vi "gds_top_tx.vi"(0 "Modulation Parameters":T2={"TX Parameters"={"Sampling Rate"=1000000.0, "Oversample Factor"=2}, "Shared Parameters"={"Packet Length"=500, "Preamble Length"=20, "modulation type"=enum."OOK", "FSK deviation (Hz)"=625.0, "Filter Parameters"={"modulation type"=enum."ASK", "pulse shaping filter (none)"=enum."none", "filter length (symbols)"=8, "filter parameter"=0.5}}}, 5 "HW parameters In":T3={"Device IP Address"="192.168.10.26", "Active Antenna"="TX1", "Carrier Frequency (Hz)"=433001000.0, "Gain (dB)"=20.0, "Generation Mode"=enum."continuous"} {"Gain (dB)" format="%.2f"; "Carrier Frequency (Hz)" format="%.2p"}, 7 "STOP":bool, 11 "error in":errorcluster) -> (1 "Transmitting":bool, 2 "coerced carrier frequency (Hz)":dbl format="%#_6p", 3 "coerced gain (dB)":dbl format="%#_6f", 4 "Modulation Parameters Out":T2, 6 "HW parameters out":T3={"Device IP Address"="192.168.11.3", "Active Antenna"="TX1", "Carrier Frequency (Hz)"=915000000.0, "Gain (dB)"=10.0, "Generation Mode"=enum."continuous"} {"Gain (dB)" format="%.2f"; "Carrier Frequency (Hz)" format="%.2p"}, 8 "key bit sequence":i8[](array[numeric])=[0, 0, 0, 0, 0, 0, 0, 0, 1, 1, 1, 0, 1, 0, 0, 1, 1, 0, 1, 1, 1, 0, 0, 1, 0, 0, 0, 1, 0, 1, 0, 0, 0, 0, 1, 0, 1, 0, 1, 1, 0, 1, 0, 0, 1, 1, 1, 1, 1, 1, 0, 1, 1, 0, 0, 1, 0, 0, 1, 0, 0, 1, 0, 1, 1, 0, 1, 1, 1, 1, 1, 1, 0, 0, 1, 0, 0, 1, 1, 0, 1, 0, 1, 0, 0, 1, 1, 0, 0, 1, 1, 0, 0, 0, 0, 0, 0, 0, 1, 1, 0, 0, 0, 1, 1, 0, 0, 1, 0, 1, 0, 0, 0, 1, 1, 0, 1, 0, 0, 1, 0, 1, 1, 1, 1, 1, 1, 1, 0, 1, 0, 0, 0, 1, 0, 1, 1, 0, 0, 0, 1, 1, 1, 0, 1, 0, 1, 1, 0, 0, 1, 0, 1, 1, 0, 0, 1, 1, 1, 1, 0, 0, 0, 1, 1, 1, 1, 1, 0, 1, 1, 1, 0, 1, 0, 0, 0, 0, 0, 1, 1, 0, 1, 0, 1, 1, 0, 1, 1, 0, 1, 1, 1, 0, 1, 1, 0, 0, 0, 0, 0, 1, 0, 1, 1, 0, 1, 0, 1, 1, 1, 1, 1, 0, 1, 0, 1, 0, 1, 0, 1, 0, 0, 0, 0, 0, 0, 1, 0, 1, 0, 0, 1, 0, 1, 0, 1, 1, 1, 1, 0, 0, 1, 0, 1, 1, 1, 0, 1, 1, 1, 0, 0, 0, 0, 0, 0, 1, 1, 1, 0, 0, 1, 1, 1, 0, 1, 0, 0, 1, 0, 0, 1, 1, 1, 1, 0, 1, 0, 1, 1, 1, 0, 1, 0, 1, 0, 0, 0, 1, 0, 0, 1, 0, 0, 0, 0, 1, 1, 0, 0, 1, 1, 1, 0, 0, 0, 0, 1, 0, 1, 1, 1, 1, 0, 1, 1, 0, 1, 1, 0, 0, 1, 1, 0, 1, 0, 0, 0, 0, 1, 1, 1, 0, 1, 1, 1, 1, 0, 0, 0, 0, 1, 1, 1, 1, 1, 1, 1, 1, 1, 0, 0, 0, 0, 0, 1, 1, 1, 1, 0, 1, 1, 1, 1, 1, 0, 0, 0, 1, 0, 1, 1, 1, 0, 0, 1, 1, 0, 0, 1, 0, 0, 0, 0, 0, 1, 0, 0, 1, 0, 1, 0, 0, 1, 1, 1, 0, 1, 1, 0, 1, 0, 0, 0, 1, 1, 1, 1, 0, 0, 1, 1, 1, 1, 1, 0, 0, 1, 1, 0, 1, 1, 0, 0, 0, 1, 0, 1, 0, 1, 0, 0, 1, 0, 0, 0, 1, 1, 1, 0, 0, 0, 1, 1, 0, 1, 1, 0, 1, 0, 1, 0, 1, 1, 1, 0, 0, 0, 1, 0, 0, 1, 1, 0, 0, 0, 1, 0, 0, 0, 1, 0, 0, 0, 0, 0, 0, 0, 0, 1, 0, 0, 0, 0, 1, 0, 0, 0, 1, 1, 0, 0, 0, 0, 1, 0, 0, 1, 1], 10 "output IQ waveform":cluster{"t0":dbl, "dt":dbl, "Y":cdb[]}, 12 "packet duration (sec)":dbl min=50000000.0 max=100000000.0 step=50000000.0 format="%#_6p", 13 "symbol rate (Hz)":dbl min=50000000.0 max=100000000.0 step=50000000.0 format="%#_6p", 14 "data symbols":cdb[](array[numeric])=[0.0+0.0i, 0.7071067811865475+0.7071067811865475i, -0.7071067811865475-0.7071067811865475i, 0.7071067811865475-0.7071067811865475i, -0.7071067811865475-0.7071067811865475i, -0.7071067811865475+0.7071067811865475i, -0.7071067811865475+0.7071067811865475i, 0.7071067811865475-0.7071067811865475i, -0.7071067811865475+0.7071067811865475i, -0.7071067811865475-0.7071067811865475i, -0.7071067811865475+0.7071067811865475i, 0.7071067811865475-0.7071067811865475i, 0.7071067811865475+0.7071067811865475i, 0.7071067811865475-0.7071067811865475i, 0.7071067811865475-0.7071067811865475i, 0.7071067811865475+0.7071067811865475i, 0.7071067811865475+0.7071067811865475i, -0.7071067811865475+0.7071067811865475i, -0.7071067811865475+0.7071067811865475i, -0.7071067811865475-0.7071067811865475i, 0.7071067811865475-0.7071067811865475i, 0.7071067811865475+0.7071067811865475i, -0.7071067811865475-0.7071067811865475i, -0.7071067811865475-0.7071067811865475i, -0.7071067811865475-0.7071067811865475i, 0.7071067811865475-0.7071067811865475i, -0.7071067811865475+0.7071067811865475i, 0.7071067811865475-0.7071067811865475i, 0.7071067811865475+0.7071067811865475i, -0.7071067811865475+0.7071067811865475i, 0.7071067811865475-0.7071067811865475i, 0.7071067811865475-0.7071067811865475i, -0.7071067811865475+0.7071067811865475i, -0.7071067811865475-0.7071067811865475i, -0.7071067811865475-0.7071067811865475i, -0.7071067811865475-0.7071067811865475i, 0.7071067811865475+0.7071067811865475i, -0.7071067811865475+0.7071067811865475i, 0.7071067811865475-0.7071067811865475i, -0.7071067811865475+0.7071067811865475i, -0.7071067811865475+0.7071067811865475i, -0.7071067811865475+0.7071067811865475i, 0.7071067811865475-0.7071067811865475i, -0.7071067811865475+0.7071067811865475i, 0.7071067811865475-0.7071067811865475i, -0.7071067811865475+0.7071067811865475i, 0.7071067811865475+0.7071067811865475i, 0.7071067811865475+0.7071067811865475i, 0.7071067811865475+0.7071067811865475i, -0.7071067811865475-0.7071067811865475i, 0.7071067811865475+0.7071067811865475i, 0.7071067811865475-0.7071067811865475i, -0.7071067811865475+0.7071067811865475i, 0.7071067811865475-0.7071067811865475i, 0.7071067811865475-0.7071067811865475i, 0.7071067811865475+0.7071067811865475i, 0.7071067811865475-0.7071067811865475i, -0.7071067811865475+0.7071067811865475i, -0.7071067811865475+0.7071067811865475i, 0.7071067811865475-0.7071067811865475i, 0.7071067811865475-0.7071067811865475i, -0.7071067811865475-0.7071067811865475i, -0.7071067811865475-0.7071067811865475i, -0.7071067811865475-0.7071067811865475i, 0.7071067811865475-0.7071067811865475i, 0.7071067811865475+0.7071067811865475i, 0.7071067811865475-0.7071067811865475i, 0.7071067811865475-0.7071067811865475i, -0.7071067811865475+0.7071067811865475i, 0.7071067811865475+0.7071067811865475i, -0.7071067811865475-0.7071067811865475i, -0.7071067811865475+0.7071067811865475i, -0.7071067811865475+0.7071067811865475i, -0.7071067811865475-0.7071067811865475i, 0.7071067811865475+0.7071067811865475i, -0.7071067811865475+0.7071067811865475i, -0.7071067811865475-0.7071067811865475i, 0.7071067811865475+0.7071067811865475i, -0.7071067811865475-0.7071067811865475i, -0.7071067811865475-0.7071067811865475i, 0.7071067811865475+0.7071067811865475i, 0.7071067811865475-0.7071067811865475i, -0.7071067811865475-0.7071067811865475i, -0.7071067811865475-0.7071067811865475i, 0.7071067811865475-0.7071067811865475i, -0.7071067811865475-0.7071067811865475i, 0.7071067811865475-0.7071067811865475i, 0.7071067811865475+0.7071067811865475i, 0.7071067811865475+0.7071067811865475i, 0.7071067811865475-0.7071067811865475i, -0.7071067811865475+0.7071067811865475i, -0.7071067811865475+0.7071067811865475i, -0.7071067811865475-0.7071067811865475i, 0.7071067811865475-0.7071067811865475i, -0.7071067811865475+0.7071067811865475i, -0.7071067811865475-0.7071067811865475i, -0.7071067811865475+0.7071067811865475i, -0.7071067811865475-0.7071067811865475i, 0.7071067811865475+0.7071067811865475i, 0.7071067811865475+0.7071067811865475i, 0.7071067811865475-0.7071067811865475i, 0.7071067811865475-0.7071067811865475i, -0.7071067811865475+0.7071067811865475i, -0.7071067811865475+0.7071067811865475i, -0.7071067811865475-0.7071067811865475i, -0.7071067811865475-0.7071067811865475i, -0.7071067811865475+0.7071067811865475i, -0.7071067811865475+0.7071067811865475i, -0.7071067811865475+0.7071067811865475i, -0.7071067811865475+0.7071067811865475i, -0.7071067811865475+0.7071067811865475i, 0.7071067811865475+0.7071067811865475i, 0.7071067811865475+0.7071067811865475i, 0.7071067811865475-0.7071067811865475i, 0.7071067811865475-0.7071067811865475i, 0.7071067811865475+0.7071067811865475i, -0.7071067811865475+0.7071067811865475i, -0.7071067811865475+0.7071067811865475i, -0.7071067811865475-0.7071067811865475i, -0.7071067811865475-0.7071067811865475i, 0.7071067811865475+0.7071067811865475i, -0.7071067811865475+0.7071067811865475i, -0.7071067811865475-0.7071067811865475i, -0.7071067811865475+0.7071067811865475i, -0.7071067811865475-0.7071067811865475i, -0.7071067811865475+0.7071067811865475i, 0.7071067811865475+0.7071067811865475i, 0.7071067811865475+0.7071067811865475i, 0.7071067811865475-0.7071067811865475i, -0.7071067811865475-0.7071067811865475i, 0.7071067811865475+0.7071067811865475i, -0.7071067811865475-0.7071067811865475i, -0.7071067811865475+0.7071067811865475i, -0.7071067811865475+0.7071067811865475i, 0.7071067811865475-0.7071067811865475i, 0.7071067811865475+0.7071067811865475i, -0.7071067811865475-0.7071067811865475i, -0.7071067811865475-0.7071067811865475i, 0.7071067811865475-0.7071067811865475i, 0.7071067811865475-0.7071067811865475i, -0.7071067811865475-0.7071067811865475i, 0.7071067811865475-0.7071067811865475i, 0.7071067811865475-0.7071067811865475i, 0.7071067811865475+0.7071067811865475i, 0.7071067811865475-0.7071067811865475i, 0.7071067811865475+0.7071067811865475i, -0.7071067811865475+0.7071067811865475i, 0.7071067811865475+0.7071067811865475i, 0.7071067811865475-0.7071067811865475i, -0.7071067811865475+0.7071067811865475i, 0.7071067811865475-0.7071067811865475i, -0.7071067811865475-0.7071067811865475i, 0.7071067811865475+0.7071067811865475i, 0.7071067811865475+0.7071067811865475i, -0.7071067811865475+0.7071067811865475i, -0.7071067811865475-0.7071067811865475i, -0.7071067811865475-0.7071067811865475i, 0.7071067811865475-0.7071067811865475i, -0.7071067811865475+0.7071067811865475i, -0.7071067811865475-0.7071067811865475i, 0.7071067811865475+0.7071067811865475i, -0.7071067811865475-0.7071067811865475i, 0.7071067811865475-0.7071067811865475i, 0.7071067811865475+0.7071067811865475i, 0.7071067811865475+0.7071067811865475i, -0.7071067811865475-0.7071067811865475i, -0.7071067811865475+0.7071067811865475i, -0.7071067811865475-0.7071067811865475i, -0.7071067811865475-0.7071067811865475i, 0.7071067811865475+0.7071067811865475i, 0.7071067811865475+0.7071067811865475i, -0.7071067811865475-0.7071067811865475i, -0.7071067811865475-0.7071067811865475i, -0.7071067811865475-0.7071067811865475i, -0.7071067811865475-0.7071067811865475i, -0.7071067811865475+0.7071067811865475i, 0.7071067811865475+0.7071067811865475i, 0.7071067811865475+0.7071067811865475i, -0.7071067811865475-0.7071067811865475i, -0.7071067811865475-0.7071067811865475i, 0.7071067811865475-0.7071067811865475i, -0.7071067811865475-0.7071067811865475i, -0.7071067811865475-0.7071067811865475i, 0.7071067811865475+0.7071067811865475i, 0.7071067811865475-0.7071067811865475i, 0.7071067811865475-0.7071067811865475i, -0.7071067811865475-0.7071067811865475i, 0.7071067811865475+0.7071067811865475i, -0.7071067811865475-0.7071067811865475i, 0.7071067811865475+0.7071067811865475i, -0.7071067811865475+0.7071067811865475i, 0.7071067811865475+0.7071067811865475i, 0.7071067811865475+0.7071067811865475i, -0.7071067811865475+0.7071067811865475i, 0.7071067811865475-0.7071067811865475i, 0.7071067811865475-0.7071067811865475i, 0.7071067811865475+0.7071067811865475i, -0.7071067811865475-0.7071067811865475i, -0.7071067811865475+0.7071067811865475i, -0.7071067811865475-0.7071067811865475i, 0.7071067811865475-0.7071067811865475i, 0.7071067811865475+0.7071067811865475i, 0.7071067811865475-0.7071067811865475i, -0.7071067811865475-0.7071067811865475i, -0.7071067811865475+0.7071067811865475i, 0.7071067811865475-0.7071067811865475i, -0.7071067811865475-0.7071067811865475i, -0.7071067811865475-0.7071067811865475i, 0.7071067811865475+0.7071067811865475i, -0.7071067811865475-0.7071067811865475i, 0.7071067811865475-0.7071067811865475i, -0.7071067811865475+0.7071067811865475i, 0.7071067811865475+0.7071067811865475i, -0.7071067811865475+0.7071067811865475i, -0.7071067811865475+0.7071067811865475i, -0.7071067811865475+0.7071067811865475i, 0.7071067811865475-0.7071067811865475i, 0.7071067811865475+0.7071067811865475i, 0.7071067811865475-0.7071067811865475i, -0.7071067811865475-0.7071067811865475i, 0.7071067811865475+0.7071067811865475i, 0.7071067811865475-0.7071067811865475i, -0.7071067811865475+0.7071067811865475i, -0.7071067811865475-0.7071067811865475i, 0.7071067811865475-0.7071067811865475i, 0.7071067811865475-0.7071067811865475i, 0.7071067811865475-0.7071067811865475i, -0.7071067811865475-0.7071067811865475i, 0.7071067811865475+0.7071067811865475i, 0.7071067811865475-0.7071067811865475i, 0.7071067811865475+0.7071067811865475i, -0.7071067811865475-0.7071067811865475i, 0.7071067811865475+0.7071067811865475i, 0.7071067811865475-0.7071067811865475i, 0.7071067811865475+0.7071067811865475i, 0.7071067811865475-0.7071067811865475i, 0.7071067811865475+0.7071067811865475i, 0.7071067811865475+0.7071067811865475i, 0.7071067811865475+0.7071067811865475i, 0.7071067811865475+0.7071067811865475i, -0.7071067811865475+0.7071067811865475i, 0.7071067811865475+0.7071067811865475i, 0.7071067811865475-0.7071067811865475i, 0.7071067811865475+0.7071067811865475i, 0.7071067811865475-0.7071067811865475i, -0.7071067811865475+0.7071067811865475i, 0.7071067811865475+0.7071067811865475i, 0.7071067811865475-0.7071067811865475i, 0.7071067811865475+0.7071067811865475i, -0.7071067811865475-0.7071067811865475i], 15 "error out":errorcluster)   [LabVIEW 2012]
uses:
  EE 497/LABS/SDR/control_type_defs.llb/tx_hw params.ctl
panel:
  in  "Configuration Out":T1(tab)
  in  "Configuration In":T1(tab)
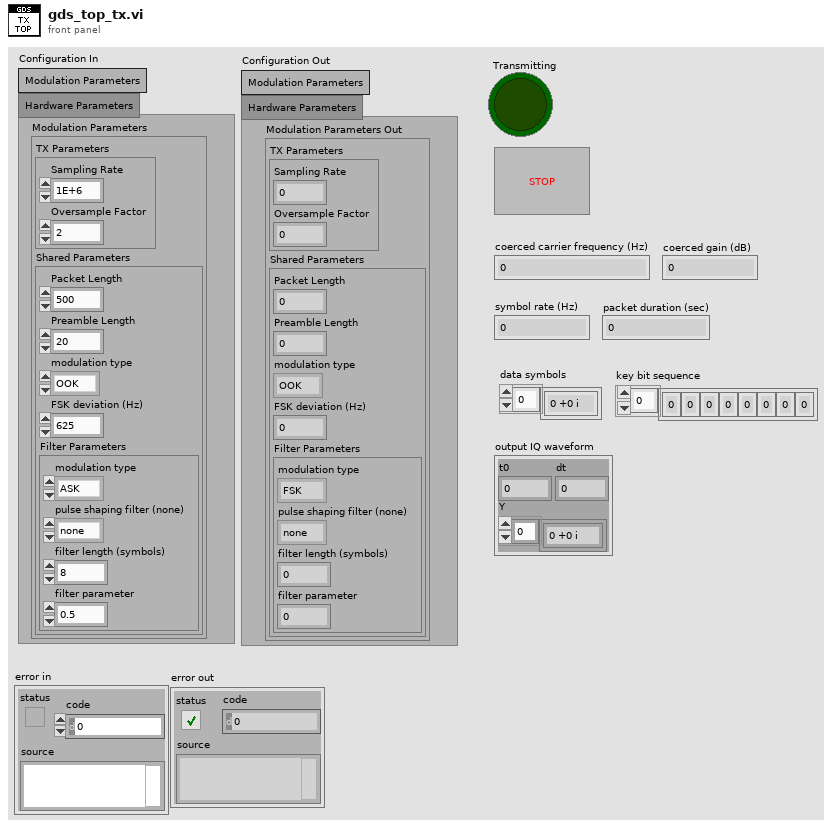
[diagram p1: front panel]
types:
  T1 = enum32{"Modulation Parameters", "Hardware Parameters"}
  T2 = cluster{"TX Parameters":cluster{"Sampling Rate":dbl, "Oversample Factor":i32}, "Shared Parameters":cluster{"Packet Length":i32, "Preamble Length":i32, "modulation type":enum16{"OOK", "FSK", "PSK", "QAM", "MSK", "PAM", "ASK", "CPM"}, "FSK deviation (Hz)":dbl, "Filter Parameters":cluster{"modulation type":enum16{"FSK", "PSK", "QAM", "MSK", "PAM", "ASK", "CPM"}, "pulse shaping filter (none)":enum16{"none", "Raised Cosine", "Root Raised Cos", "Gaussian"}, "filter length (symbols)":i32, "filter parameter":dbl}}}
  T3 = typedef "tx_hw params.ctl" = cluster{"Device IP Address":refnum<k15>, "Active Antenna":string, "Carrier Frequency (Hz)":dbl, "Gain (dB)":dbl, "Generation Mode":enum16{"single shot", "simulate", "continuous"}}
  T4 = typedef "niAMT.lvlib/Complex Data Waveform.ctl" = cluster{"t0":dbl, "dt":dbl, "Y":cdb[]}
  T5 = cluster{"Sampling Rate":dbl, "Oversample Factor":i32}
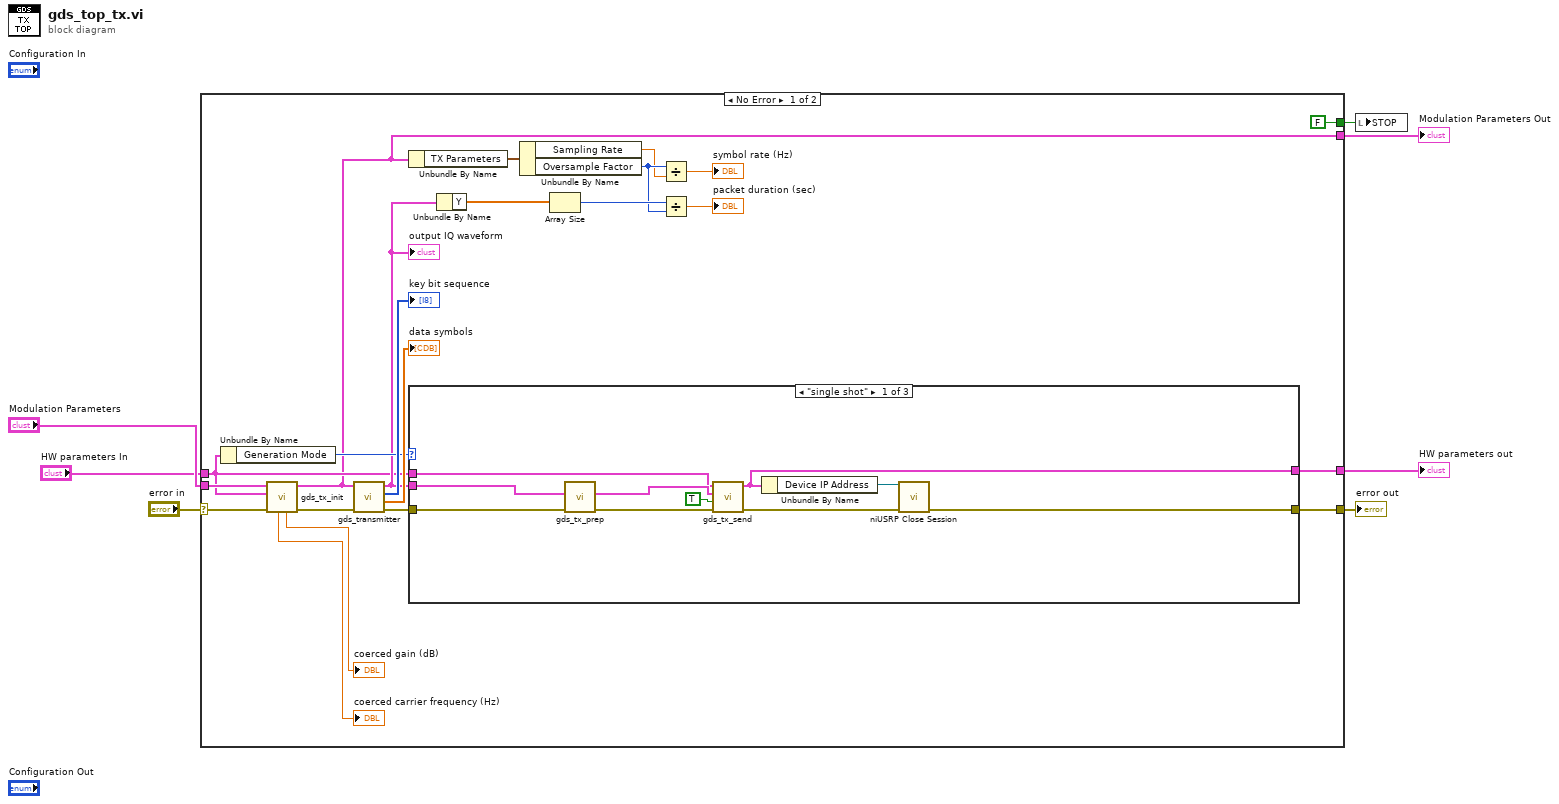
[diagram p0: block diagram]
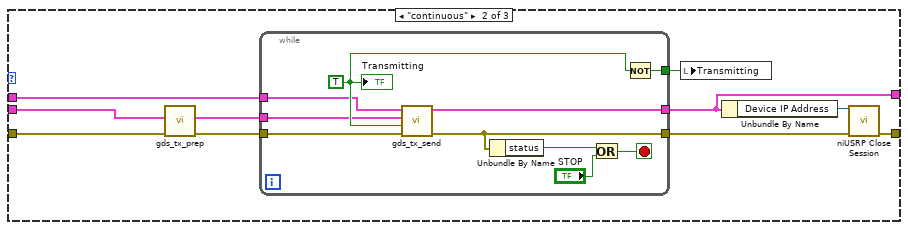
[diagram p2: hidden frame]
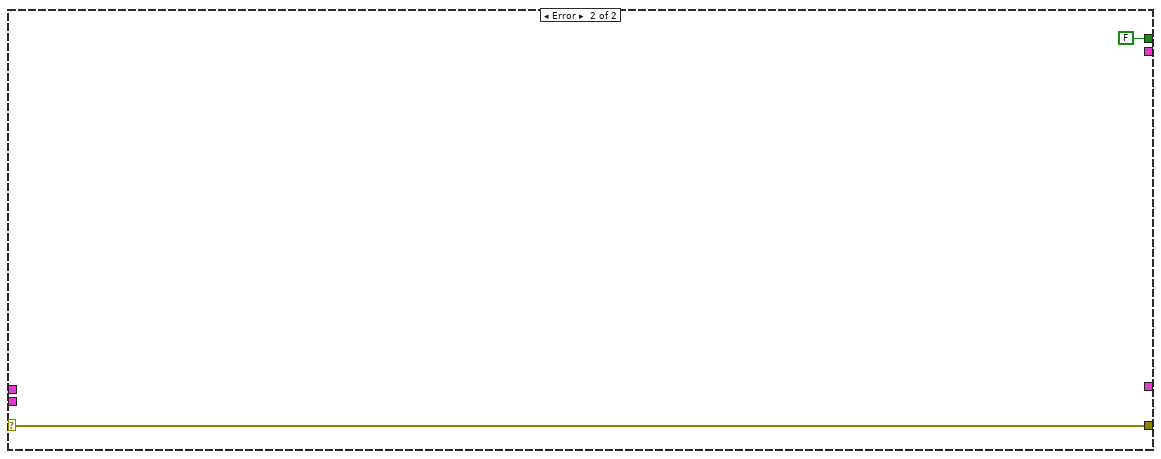
[diagram p4: hidden frame]
diagram:
  n1 = case shown="No Error" "error in" {
    selector: "error in" -> [w27 w62]
    tunnel: "Modulation Parameters" -> [w11 _]
    tunnel: "HW parameters In" -> [w10 _]
    tunnel: [FALSE FALSE ("Done")] -> w6
    tunnel: [w13 w62] -> w5
    tunnel: [w9 _] -> w2
    tunnel: [w8 _] -> w1
    frame No Error {
      n2 = Unbundle By Name(w10) -> ("Generation Mode"=w15:enum16{"single shot", "simulate", "continuous"})
      n3 = call "gds_tx_init.vi"("error in (no error)"=w27, "HW parameters In"=w10, "Modulation Parameters"=w11) -> ("error out"=w26:errorcluster, "Modulation Parameters Out"=w8:T2, "coerced gain (dB)"=→"coerced gain (dB)":dbl, "coerced carrier frequency (Hz)"=→"coerced carrier frequency (Hz)":dbl)  [unwired: 4 in, 1 out]
      n4 = call "gds_transmitter.vi"("error in (no error)"=w26, "Modulation Parameters"=w8) -> ("error out"=w14:errorcluster, "Symbols Out"=→"data symbols":cdb[], "Key Bit Sequence"=→"key bit sequence":i8[], "Transmitted Signal"=w12:T4)  [unwired: 6 in]
      "output IQ waveform" <- w12
      n5 = Unbundle By Name(w8) -> ("TX Parameters"=w23:T5)
      n6 = case shown="\"single shot\"" w15 {
        tunnel: w12 -> [w39 w49 _]
        tunnel: w14 -> [w38 w48 w61]
        tunnel: [w37 w44 w61] -> w13
        tunnel: w10 -> [w31 w41 w60]
        tunnel: [w30 w40 w60] -> w9
        frame "single shot" {
          n7 = call "gds_tx_prep.vi"("error in (no error)"=w38, "input IQ waveform"=w39) -> ("error out"=w35:errorcluster, "Scaled and Padded IQ waveform"=w34:cluster{"t0":dbl, "dt":dbl, "Y":cdb[]})  [unwired: 8 in]
          n8 = call "gds_tx_send.vi"("error in (no error)"=w35, "end of data?"=TRUE, "IQ Data in"=w34, "HW parameters in"=w31) -> ("error out"=w36:errorcluster, "HW parameters out"=w30:T3)  [unwired: 6 in]
          n9 = Unbundle By Name(w30) -> ("Device IP Address"=w33:refnum<k15>)
          n10 = call <instrlib>:"niUSRP Close Session.vi"("session handle"=w33, "error in (no error)"=w36) -> ("error out"=w37:errorcluster)  [unwired: 13 in]
        }
        frame "continuous" {
          n11 = call "gds_tx_prep.vi"("error in (no error)"=w48, "input IQ waveform"=w49) -> ("error out"=w47:errorcluster, "Scaled and Padded IQ waveform"=w43:cluster{"t0":dbl, "dt":dbl, "Y":cdb[]})  [unwired: 8 in]
          n12 = while {
            tunnel: w47 -> [w59]
            tunnel: [w55] -> w46
            tunnel: [w54] -> w45
            tunnel: w43 -> [w52]
            tunnel: [w51] -> w40
            tunnel: w41 -> [w50]
            stop <- w56 stop-if-true
            w53 = TRUE
            n13 = call "gds_tx_send.vi"("error in (no error)"=w59, "end of data?"=w53, "IQ Data in"=w52, "HW parameters in"=w50) -> ("error out"=w54:errorcluster, "HW parameters out"=w51:T3)  [unwired: 6 in]
            n14 = Unbundle By Name(w54) -> ("status"=w58:bool)
            n15 = Or(x=w58, y="STOP") -> (x .or. y?=w56:bool)
            n16 = Not(x=w53) -> (.not. x?=w55:bool)
            "Transmitting" <- w53
          }
          n17 = local write "Transmitting"(w46) -> ()
          n18 = Unbundle By Name(w40) -> ("Device IP Address"=w42:refnum<k15>)
          n19 = call <instrlib>:"niUSRP Close Session.vi"("session handle"=w42, "error in (no error)"=w45) -> ("error out"=w44:errorcluster)  [unwired: 13 in]
        }
        frame "simulate", Default {
        }
      }
      n20 = Unbundle By Name(w12) -> ("Y"=w22:cdb[])
      n21 = Unbundle By Name(w23) -> ("Sampling Rate"=w19:dbl, "Oversample Factor"=w20:i32)
      n22 = Array Size(array=w22) -> (size(s)=w21:i32)
      n23 = Divide(x=w20, y=w19) -> (x/y=→"symbol rate (Hz)":dbl)
      n24 = Divide(x=w21, y=w20) -> (x/y=→"packet duration (sec)":dbl)
    }
    frame Error {
    }
  }
  "error out" <- w5
  "HW parameters out" <- w2
  "Modulation Parameters Out" <- w1
  n25 = local write "STOP"(w6) -> ()
